vi "Read NmdNumericSize.vi"(9 "NamedNumeric in":refnum<class "NamedNumeric.lvclass">) -> (3 "NamedNumeric out":refnum<class "NamedNumeric.lvclass">, 4 "NmdNumericSize":T1)   [LabVIEW 2014, in "Raspberry Pi Compatible Compiler for LabVIEW.lvlib" / "NamedNumeric.lvclass"]
uses:
  NamedNumeric.lvclass
  <vilib>/Utility/miscctls.llb/LVBoundsTypeDef.ctl
  NamedNumeric.lvclass/NamedNumeric.ctl
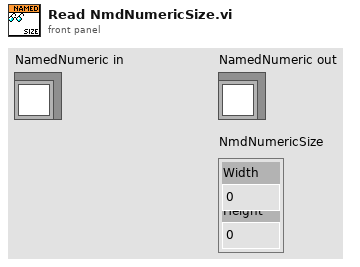
[diagram p1: front panel]
types:
  T1 = typedef "LVBoundsTypeDef.ctl" = cluster{"Width":u32, "Height":u32}
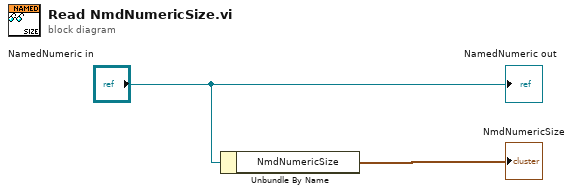
[diagram p0: block diagram]
diagram:
  n1 = Unbundle By Name("NamedNumeric in") -> ("NmdNumericSize"=→"NmdNumericSize":T1)
  "NamedNumeric out" <- "NamedNumeric in"
